vi "Pi_Typing.vi"(8 "Update":bool, 11 "Cluster":T2) -> (1 "Script?":bool, 2 "key":string, 3 "string":string)   [LabVIEW 2019]
uses:
  <vilib>/event_ctls.llb/eventvkey.ctl
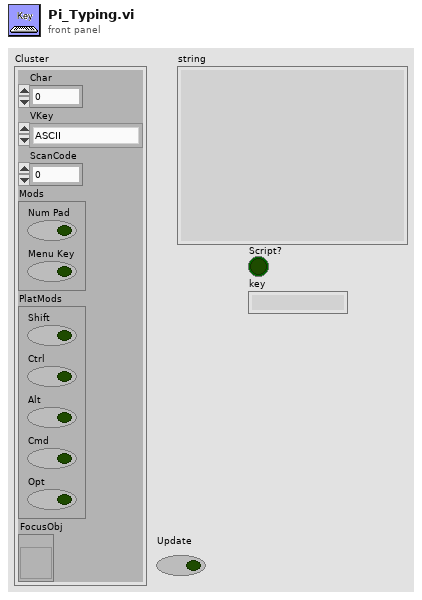
[diagram p1: front panel]
types:
  T1 = typedef "eventvkey.ctl" = enum16{"ASCII", "Enter", "Return", "Shift", "Ctrl", "Alt", "Cmd", "Opt", "Caps", "NumLock", "Clear", "Break", "Up", "Down", "Left", "Right", "Insert", "Delete", "Home", "End", "PageUp", "PageDown", "Escape", "Help", "Pause", "ScrollLock", "F1", "F2", "F3", "F4", "F5", "F6", "F7", "F8", "F9", "F10", "F11", "F12", "F13", "F14", "F15", "F16", "F17", "F18", "F19", "F20", "F21", "F22", "F23", "F24", "Play", "VolumeUp", "VolumeDown", "Mute", "Two Byte Char"}
  T2 = cluster{"Char":i16, "VKey":T1, "ScanCode":i16, "Mods":cluster{"Num Pad":bool, "Menu Key":bool}, "PlatMods":cluster{"Shift":bool, "Ctrl":bool, "Alt":bool, "Cmd":bool, "Opt":bool}, "FocusObj":refnum<vi>}
  T3 = cluster{"Shift":bool, "Ctrl":bool, "Alt":bool, "Cmd":bool, "Opt":bool}
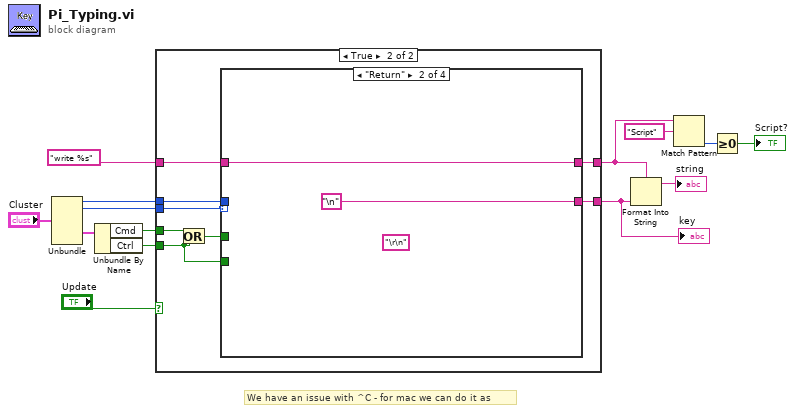
[diagram p0: block diagram]
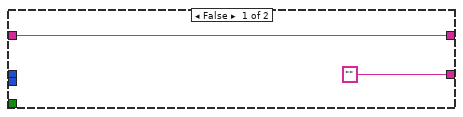
[diagram p2: hidden frame]
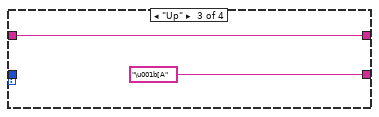
[diagram p4: hidden frame]
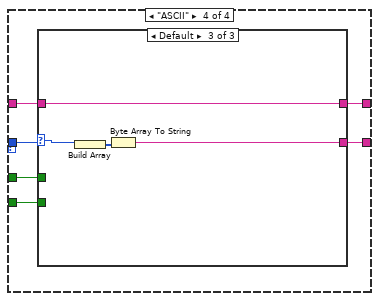
[diagram p5: hidden frame]
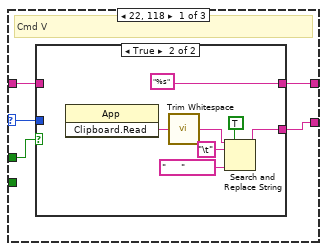
[diagram p6: hidden frame]
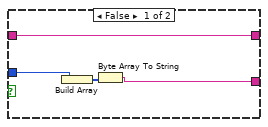
[diagram p7: hidden frame]
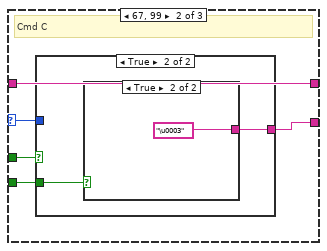
[diagram p8: hidden frame]
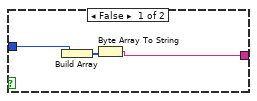
[diagram p9: hidden frame]
diagram:
  # "We have an issue with ^C - for mac we can do it as"
  n1 = Unbundle("Cluster") -> ("Char"=w13:i16, "VKey"=w12:T1, "PlatMods"=w11:T3)  [unwired: 3 out]
  n2 = Unbundle By Name(w11) -> ("Cmd"=w7:bool, "Ctrl"=w10:bool)
  n3 = case shown="True" "Update" {
    tunnel: ["" ("string") w24] -> w9
    tunnel: w13 -> [_ w23]
    tunnel: w12 -> [_ w22]
    tunnel: w10 -> [_ w19]
    tunnel: w7 -> [_ w20]
    tunnel: [w15 w18] -> w5
    tunnel: "write %s" -> [w15 w17]
    frame False {
    }
    frame True {
      n4 = Or(x=w20, y=w19) -> (x .or. y?=w21:bool)
      n5 = case shown="\"Return\"" w22 {
        tunnel: [_ "\n" ("string") "\u001b[A" ("string") w35] -> w24
        tunnel: w23 -> [_ _ _ w34]
        tunnel: w21 -> [_ _ _ w33]
        tunnel: w19 -> [_ _ _ w32]
        tunnel: [w25 w26 w28 w31] -> w18
        tunnel: w17 -> [w25 w26 w28 w30]
        frame Default {
        }
        frame "Return" {
          (unwired) "\r\n" ("string")
        }
        frame "Up" {
        }
        frame "ASCII" {
          n6 = case shown="Default" w34 {
            selector: w34 -> [w38 w54 w64]
            tunnel: [w40 w56 w66] -> w35
            tunnel: w33 -> [w39 w55 _]
            tunnel: w32 -> [_ w53 _]
            tunnel: [w37 w52 w63] -> w31
            tunnel: w30 -> [w36 w52 w63]
            frame 22, 118 {
              # "Cmd V"
              n7 = case shown="True" w39 {
                tunnel: [w42 w46] -> w40
                tunnel: w38 -> [w43 _]
                tunnel: [w41 "%s"] -> w37
                tunnel: w36 -> [w41 _]
                frame False {
                  n8 = Build Array(w43) -> (w44:i16[])
                  n9 = Byte Array To String(unsigned byte array=w44) -> (string=w42:string)
                }
                frame True {
                  n10 = invoke class="App" method="Clipboard.Read"() -> ("Read Clipbrd"=w51:string)  [unwired: 3 in, 2 out]
                  n11 = call <vilib>:"Trim Whitespace.vi"("string"=w51) -> ("trimmed string"=w50:string)  [unwired: 1 in]
                  n12 = Search and Replace String(replace all?=TRUE ("replace all? (F)"), input string=w50, search string="\t", replace string="     " ("replace string (\"\")")) -> (result string=w46:string)  [unwired: 4 in, 3 out]
                }
              }
            }
            frame 67, 99 {
              # "Cmd C"
              n13 = case shown="True" w55 {
                tunnel: [w57 w60] -> w56
                tunnel: w54 -> [w58 _]
                tunnel: w53 -> [_ w61]
                frame False {
                  n14 = Build Array(w58) -> (w59:i16[])
                  n15 = Byte Array To String(unsigned byte array=w59) -> (string=w57:string)
                }
                frame True {
                  n16 = case shown="True" w61 {
                    tunnel: [_ "\u0003"] -> w60
                    frame False {
                    }
                    frame True {
                    }
                  }
                }
              }
            }
            frame Default {
              n17 = Build Array(w64) -> (w65:i16[])
              n18 = Byte Array To String(unsigned byte array=w65) -> (string=w66:string)
            }
          }
        }
      }
    }
  }
  "key" <- w9
  n19 = Format Into String(format string=w5, w9) -> (resulting string=→"string":string)  [unwired: 2 in, 1 out]
  n20 = Match Pattern(string=w5, regular expression="Script") -> (offset past match=w3:i32)  [unwired: 1 in, 3 out]
  n21 = Greater Or Equal To 0?(x=w3) -> (x >= 0?=→"Script?":bool)
